vi "VI Tree - LUT.vi"   [LabVIEW 2017]
uses:
  LUT.lvclass
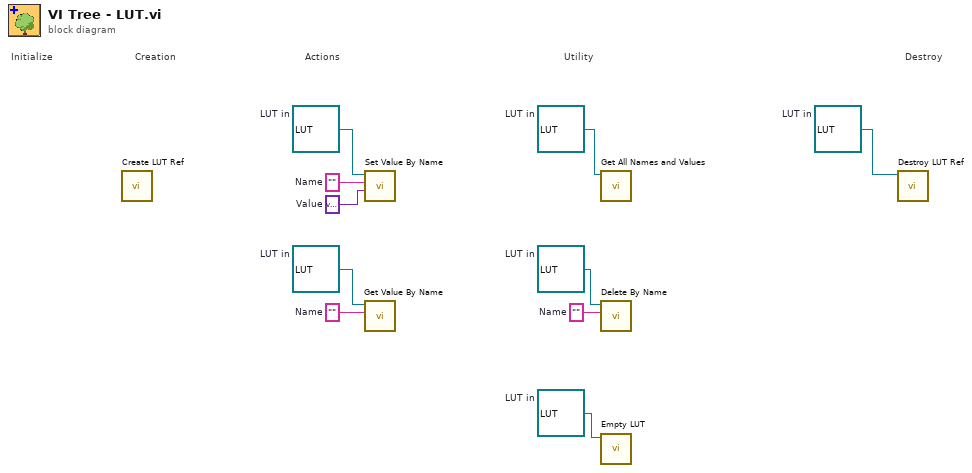
[diagram p0: block diagram]
diagram:
  w1 = refnum<class "LUT.lvclass"> refnum  # LUT in
  w2 = refnum<class "LUT.lvclass"> refnum  # LUT in
  w3 = refnum<class "LUT.lvclass"> refnum  # LUT in
  w4 = ""  # Name
  w5 = refnum<class "LUT.lvclass"> refnum  # LUT in
  w6 = refnum<class "LUT.lvclass"> refnum  # LUT in
  w7 = ""  # Name
  w8 = refnum<class "LUT.lvclass"> refnum  # LUT in
  w9 = ""  # Name
  w10 = variant  # Value
  # "Creation"
  # "Utility"
  # "Actions"
  # "Destroy"
  # "Initialize"
  n1 = call "Create LUT Ref.vi"() -> ()  [unwired: 10 in, 2 out]
  n2 = call "Set Value By Name.vi"("Value"=w10, "Name"=w9, "LUT in"=w8) -> ()  [unwired: 6 in, 3 out]
  n3 = call "Get Value By Name.vi"("Name"=w7, "LUT in"=w6) -> ()  [unwired: 6 in, 4 out]
  n4 = call "Get All Names and Values.vi"("LUT in"=w5) -> ()  [unwired: 7 in, 4 out]
  n5 = call "Delete By Name.vi"("Name"=w4, "LUT in"=w3) -> ()  [unwired: 7 in, 3 out]
  n6 = call "Empty LUT.vi"("LUT in"=w2) -> ()  [unwired: 9 in, 2 out]
  n7 = call "Destroy LUT Ref.vi"("LUT in"=w1) -> ()  [unwired: 10 in, 1 out]
